vi "tau to tw (SubVI).vi"(4 "no of R points":i32=2000, 5 "Cinf":dbl=1.0, 6 "no of C(t) points":i32=10000, 7 "C0":dbl=-1.0, 9 "polynomial order":i32=6, 10 "Phase shift":dbl=180.0 format="%#_13g", 11 "tau":dbl[unit]) -> (2 "R(t_w)":dbl, 3 "t_w":dbl[unit])   [LabVIEW 2019]
doc: "Analyzes system response for given emission time constant, calculates lock-in period and scaling factor"
uses:
  <vilib>/Analysis/polynomials.llb/nth Derivative of Polynomial (DBL).vi
  <vilib>/Analysis/polynomials.llb/Polynomial Roots (DBL).vi
  <vilib>/Analysis/polynomials.llb/Scalar Polynomial Evaluation (DBL).vi
  <vilib>/Analysis/NI_AALPro.lvlib
  <vilib>/Analysis/NI_AALBase.lvlib
panel:
  out "standard deviation":dbl format="%.7f"
  out "Polynomial Coefficients":dbl[](array[numeric])
  out "tau/t_w":dbl
  out "Scan Results":cluster{dbl[], "Best Polynomial Fit":dbl[]}[](graph)
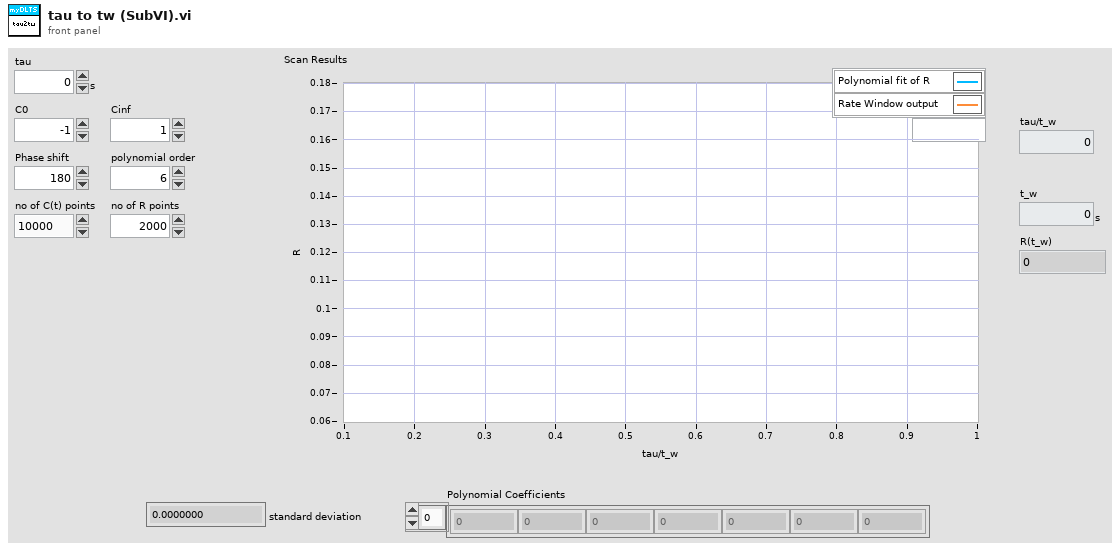
[diagram p1: front panel]
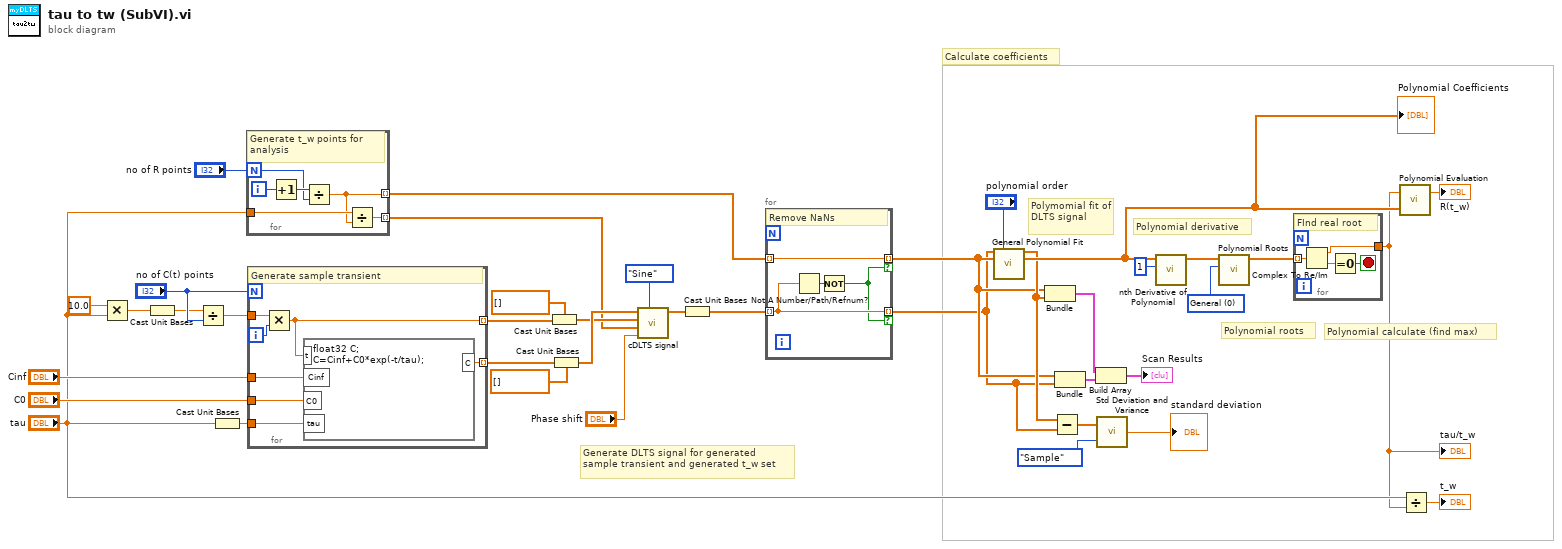
[diagram p0: block diagram]
diagram:
  w22 = u16 0 items=["General", "Simple Classification", "Refinement", "Advanced Refinement"] ("option")
  # "Calculate coefficients"
  # "Polynomial calculate (find max)"
  # "Polynomial roots"
  # "Polynomial derivative"
  # "Polymomial fit of DLTS signal"
  # "Generate DLTS signal for generated sample transient and generated t_w set"
  n1 = Multiply(x=10.0, y="tau") -> (x*y=w31:dbl[unit])
  n2 = Cast Unit Bases(0:w31) -> (2:w9:dbl)  [unwired: 1 in]
  n3 = Divide(x=w9, y="no of C(t) points") -> (x/y=w12:dbl)
  n4 = Cast Unit Bases(0:"tau") -> (2:w10:dbl)  [unwired: 1 in]
  n5 = for {
    N: "no of R points" -> [w41]
    tunnel: "tau" -> [w44]
    tunnel: [w43] -> w26 mode=indexing
    tunnel: [w42] -> w8 mode=indexing
    i -> [w46]
    # "Generate t_w points for analysis"
    n6 = Increment(x=w46) -> (x+1=w45:i32)
    n7 = Divide(x=w45, y=w41) -> (x/y=w43:dbl)
    n8 = Divide(x=w44, y=w43) -> (x/y=w42:dbl[unit])
  }
  n9 = for {
    N: "no of C(t) points" -> [_]
    tunnel: w12 -> [w52]
    tunnel: [w51] -> w36 mode=indexing
    tunnel: w10 -> [w50]
    tunnel: "C0" -> [w49]
    tunnel: "Cinf" -> [w48]
    tunnel: [w47] -> w13 mode=indexing
    i -> [w53]
    # "Generate sample transient"
    n10 = Multiply(x=w52, y=w53) -> (x*y=w51:dbl)
    n11 = formula code="float32 C;\nC=Cinf+C0*exp(-t/tau);"("C0"=w49, "tau"=w50, "t"=w51, "Cinf"=w48) -> ("C"=w47:sgl)
  }
  n12 = Cast Unit Bases(0:w36, 1:dbl[unit][] [] ("t")) -> (2:w34:dbl[unit][])
  n13 = Cast Unit Bases(0:w13, 1:dbl[unit][] [] ("C(t)")) -> (2:w37:sgl[unit][])
  n14 = call "cDLTS signal.vi"("Weight function"=enum16{"Square", "Sine"}."Sine", "Phase shift"="Phase shift", "t_w"=w8, "t"=w34, "C(t)"=w37) -> ("S"=w27:dbl[unit][])  [unwired: 4 in]
  n15 = Cast Unit Bases(0:w27) -> (2:w6:dbl[])  [unwired: 1 in]
  n16 = for {
    tunnel: w6 -> [w55] mode=indexing
    tunnel: w26 -> [w57] mode=indexing
    tunnel: [w57] -> w2 mode=indexing if=w54
    tunnel: [w55] -> w1 mode=indexing if=w54
    # "Remove NaNs"
    n17 = Not A Number/Path/Refnum?(number/path/refnum=w55) -> (NaN/Path/Refnum?=w56:bool)
    n18 = Not(x=w56) -> (.not. x?=w54:bool)
  }
  n19 = call <vilib>:"General Polynomial Fit.vi"("Y"=w1, "polynomial order"="polynomial order", "X"=w2) -> ("Best Polynomial Fit"=w7:dbl[], "Polynomial Coefficients"=w19:dbl[])  [unwired: 9 in, 2 out]
  "Polynomial Coefficients" <- w19
  n20 = Bundle(w2, "Best Polynomial Fit"=w7) -> (w24:cluster{dbl[], "Best Polynomial Fit":dbl[]})  [unwired: 1 in]
  n21 = Subtract(x=w7, y=w1) -> (x-y=w5:dbl[])
  n22 = Bundle(w2, w1) -> (w29:cluster{dbl[], dbl[]})  [unwired: 1 in]
  n23 = Build Array(w24, w29) -> (→"Scan Results":cluster{dbl[], "Best Polynomial Fit":dbl[]}[])
  n24 = call <vilib>:"Std Deviation and Variance.vi"("X"=w5, "Weighting (Sample)"=enum16{"Sample", "Population"}."Sample") -> ("standard deviation"=→"standard deviation":dbl)  [unwired: 2 out]
  n25 = call-poly <vilib>:"nth Derivative of Polynomial.vi"("order"=1, "P(x)"=w19) -> ("Nth Derivative of P(x)"=w20:dbl[])  [unwired: 8 in, 1 out]
  n26 = call-poly <vilib>:"Polynomial Roots.vi"("option"=w22, "P(x)"=w20) -> ("Roots"=w21:cdb[])  [unwired: 8 in, 1 out]
  n27 = for {
    tunnel: w21 -> [w61] mode=indexing
    tunnel: [w58] -> w15
    stop <- w59 stop-if-true
    # "FInd real root"
    n28 = Complex To Re/Im(x + iy=w61) -> (x=w58:dbl, y=w60:dbl)
    n29 = Equal To 0?(x=w60) -> (x = 0?=w59:bool)
  }
  "tau/t_w" <- w15
  n30 = call-poly <vilib>:"Polynomial Evaluation.vi"("P(x)"=w19, "a"=w15) -> ("P(a)"=→"R(t_w)":dbl)  [unwired: 1 out]
  n31 = Divide(x="tau", y=w15) -> (x/y=→"t_w":dbl[unit])
